vi "Sinewave_Linearity_trial_F027.vi"(0 "Array":u32[](array[numeric]), 1 "Histogram Capture Method":bool, 2 "L code":u32, 3 "UCode":dbl, 4 "Resolution":i64, 5 "Histogram: h(x)":i32[](array[numeric])) -> (6 "Average Hits \nper Code":dbl format="%.2f", 7 "Max\nDNL":dbl format="%.2f", 8 "Min\nDNL":dbl format="%.2f", 9 "Max\nINL":dbl format="%.2f", 10 "Min\nINL":dbl format="%.2f", 11 "Missing Codes":i32[](array[numeric]), 12 "Max  DNL Loc.":i32[](array[numeric]), 13 "Min DNL Loc.":i32[](array[numeric]), 14 "Max  INL Loc":i32[](array[numeric]), 15 "Min INL Loc":i32[](array[numeric]), 16 "Histogram Plot":dbl[][](graph), 17 "DNL Plot":dbl[](graph), 18 "INL Plot":dbl[](graph))   [LabVIEW 2021]
uses:
  <vilib>/Analysis/baseanly.llb/Mean (DBL).vi
  <vilib>/Analysis/NI_AALBase.lvlib
panel:
  out "range":dbl
  out "Histogram 2":dbl[](graph)
  out "2^x":dbl
  out "UCode 2":dbl
  out "L code 2":u32
  out "PI/Total no of sample":dbl
  in  "Ramp/Sine":bool
  out "Histogram raw data":i32[](graph)
  in  "Tab Control":enum32{"Histogram", "INL and DNL"}(tab)
  out "Histogram":i32[](graph)
  in  "?":bool=TRUE
  in  "?":bool
  in  "Help":bool
  in  "?":bool
  in  "file path":path
  in  "error in (not an error)":errorcluster
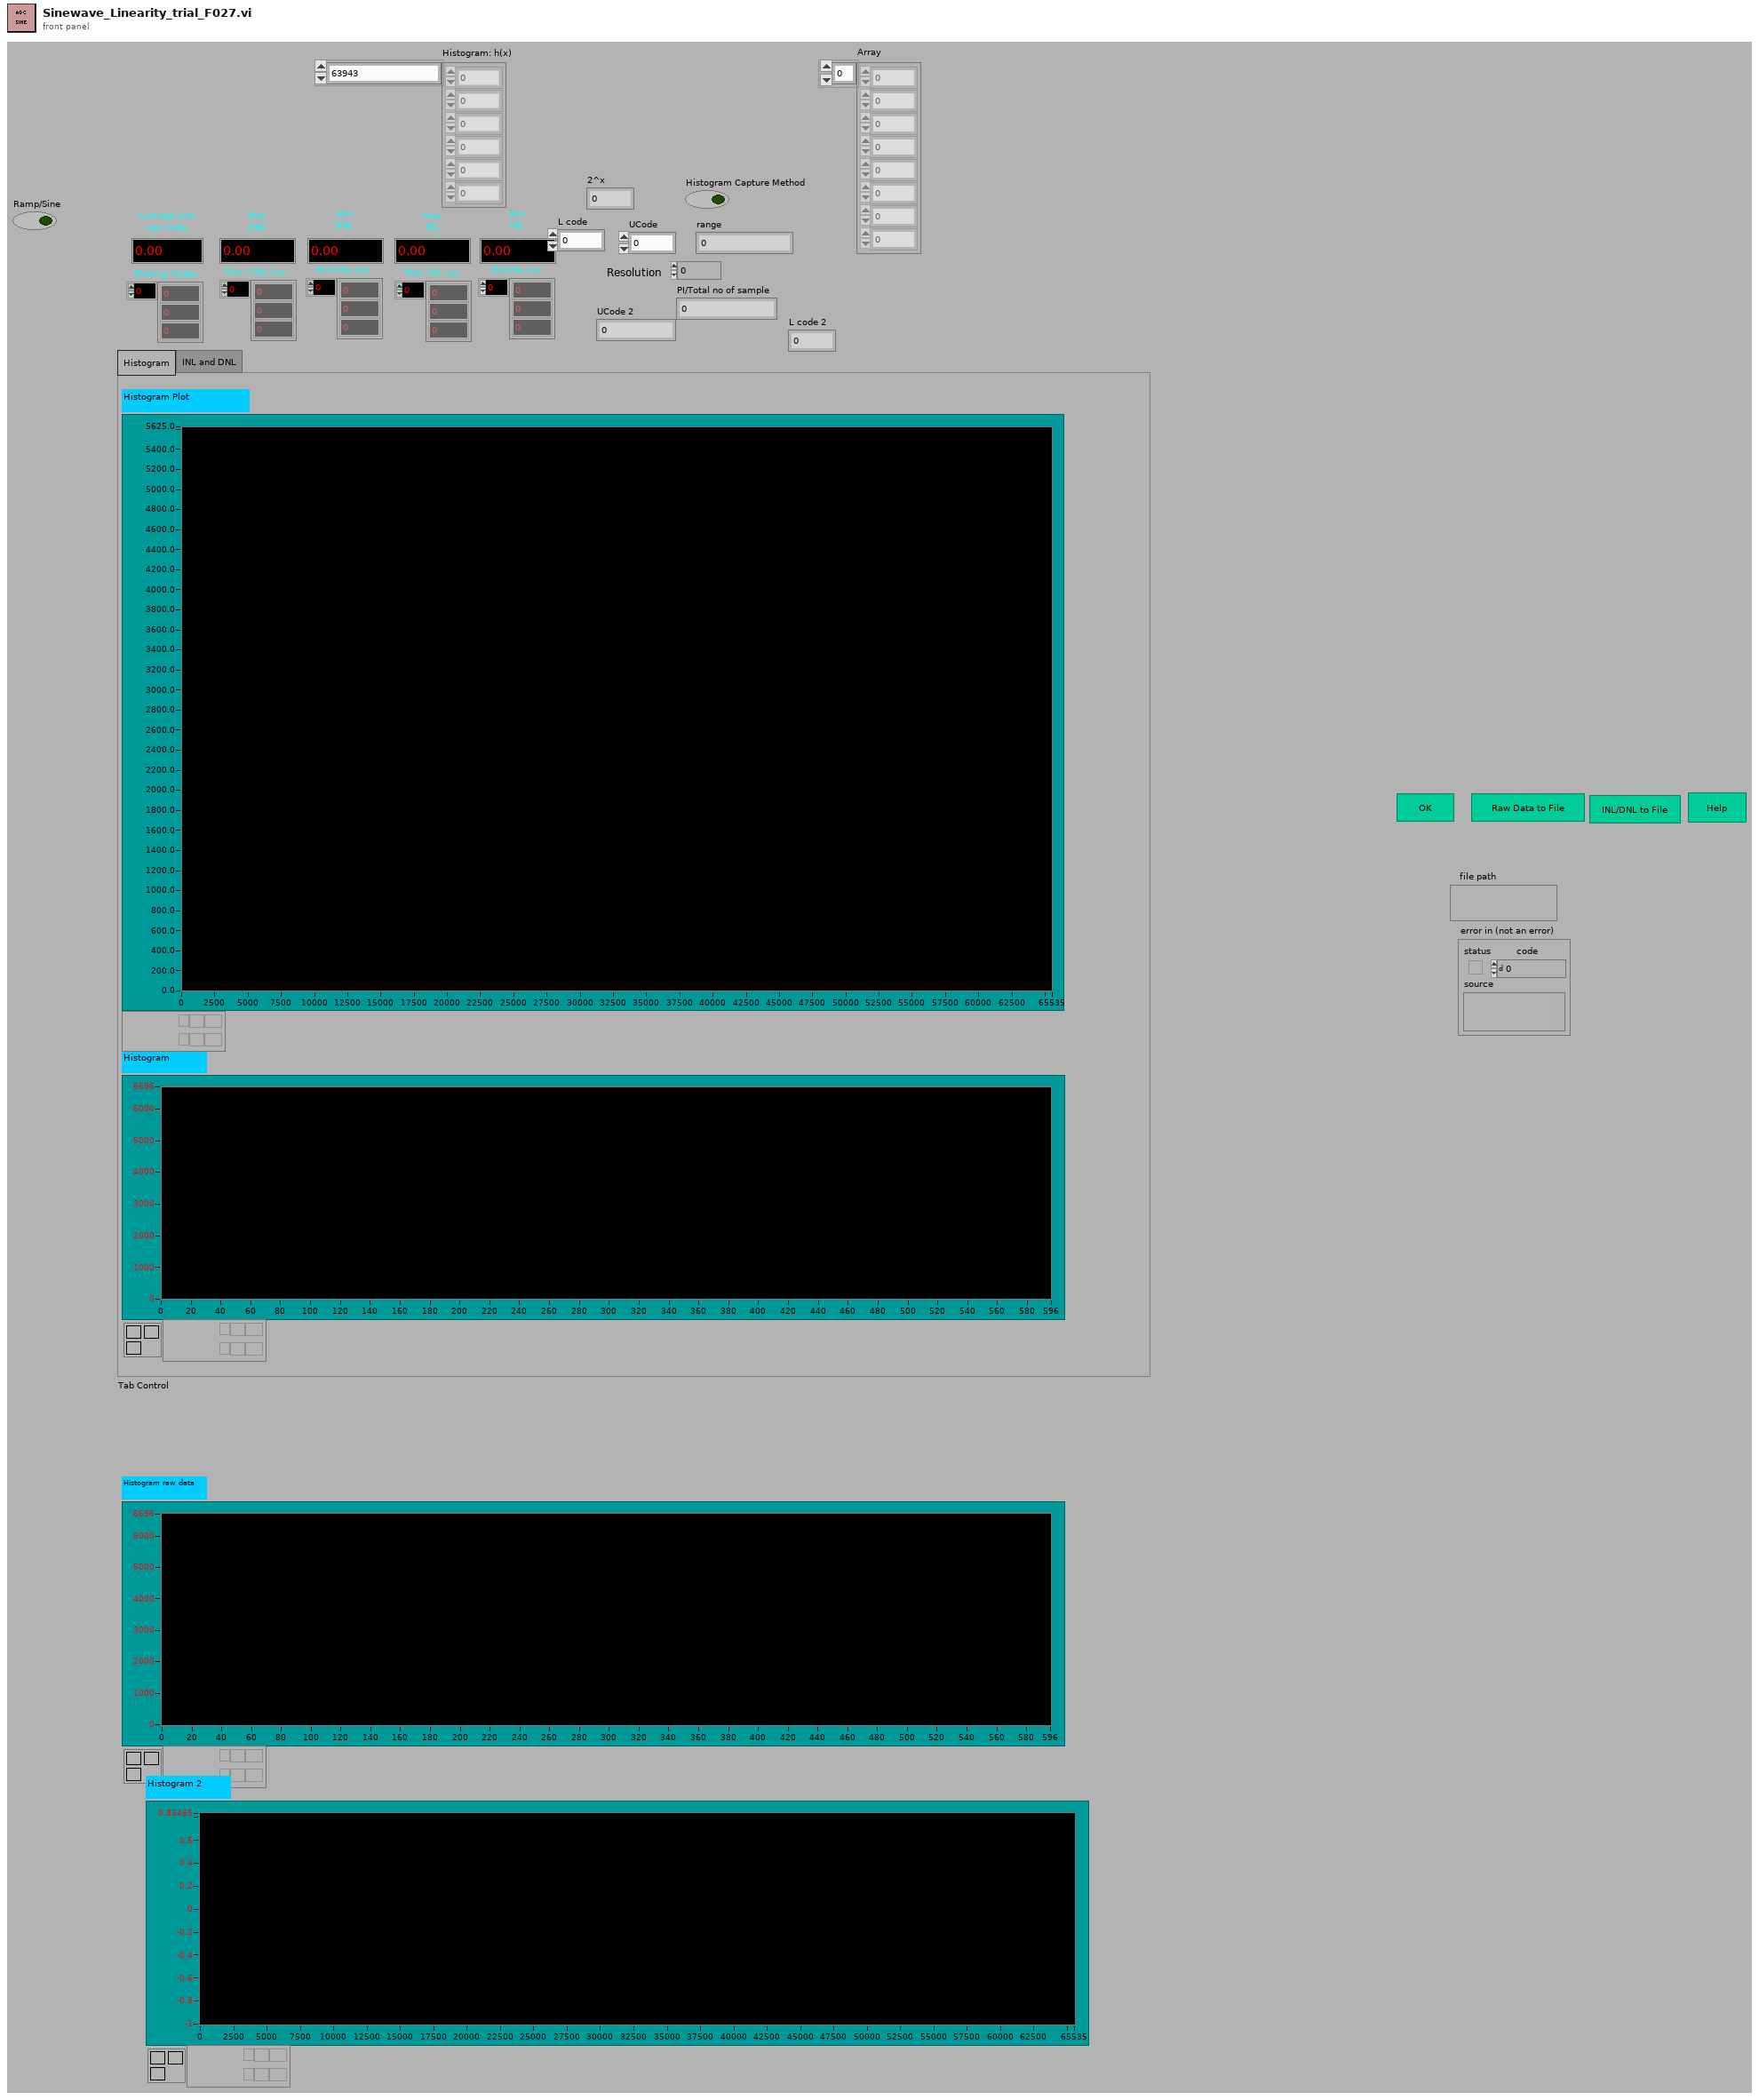
[diagram p1: front panel]
types:
  T1 = enum16{"open", "open or create", "create or replace", "create"}
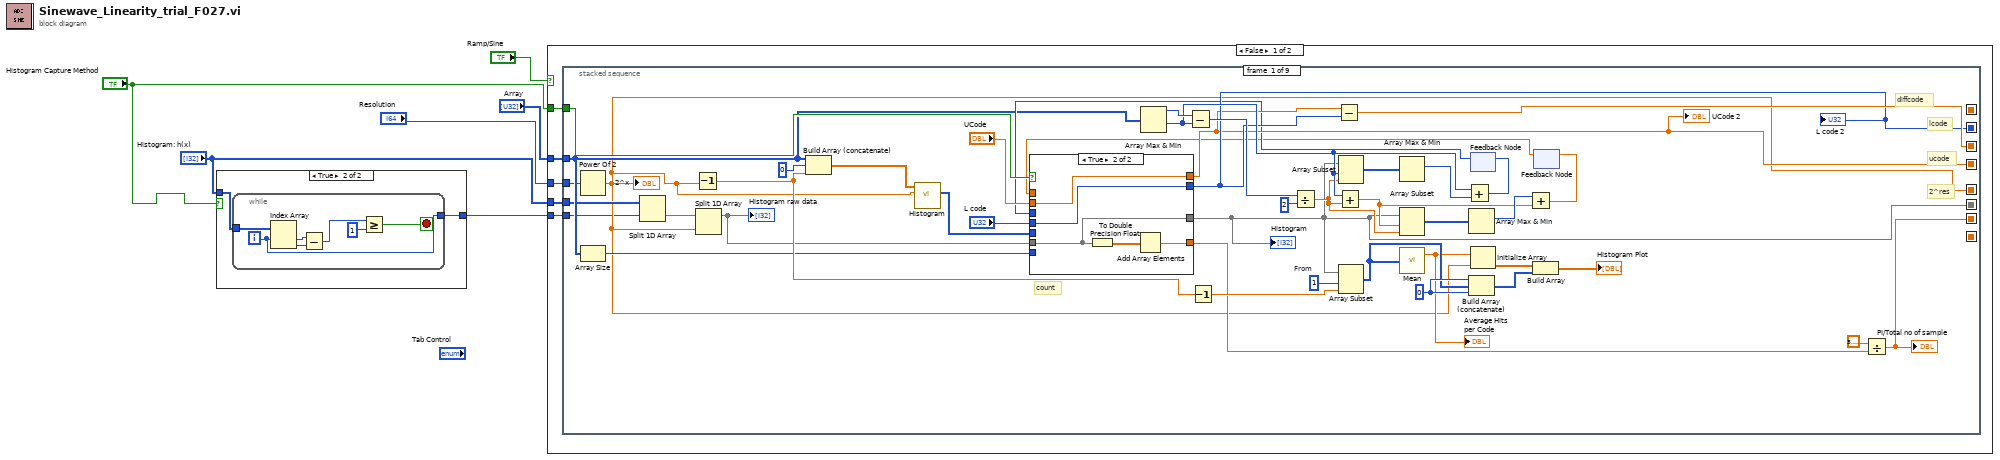
[diagram p0: block diagram]
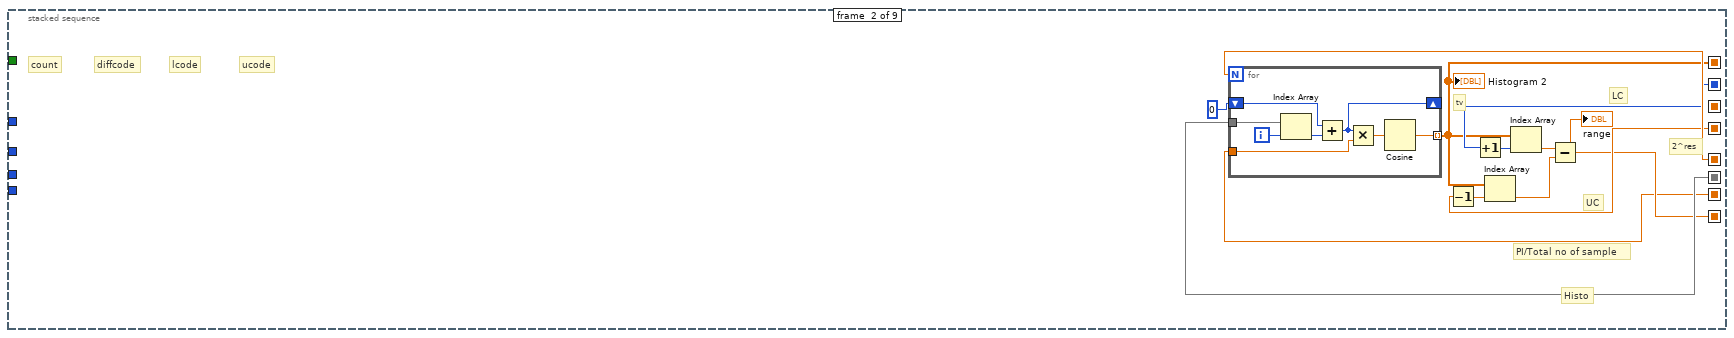
[diagram p4: hidden frame]
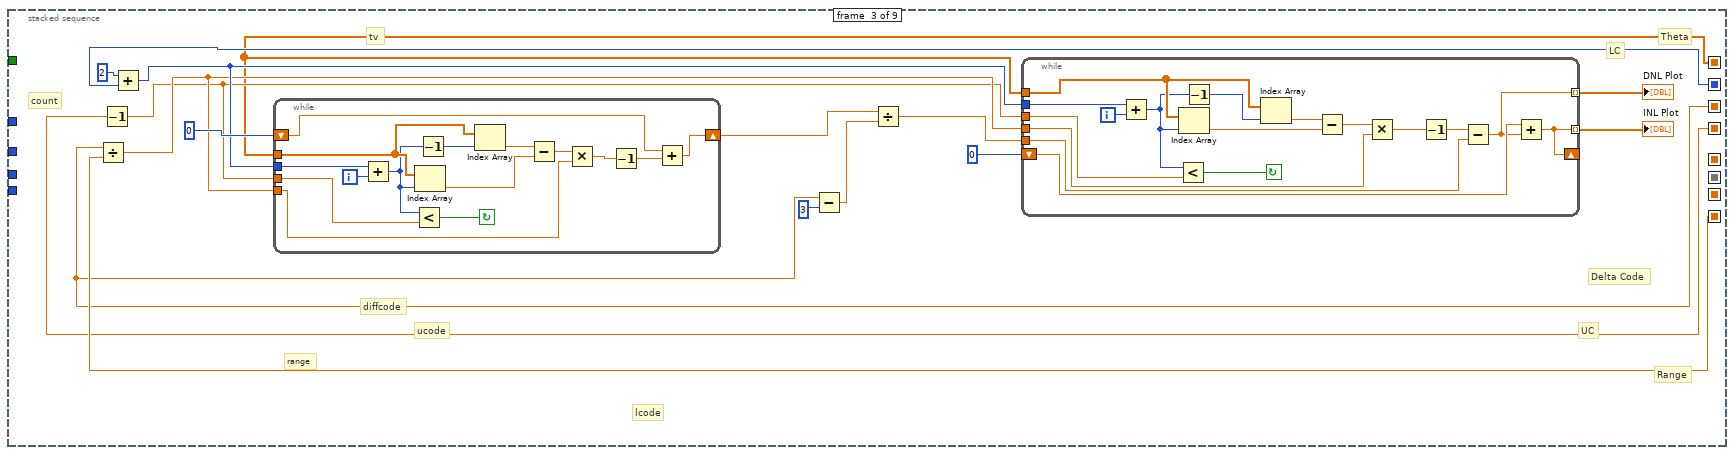
[diagram p5: hidden frame]
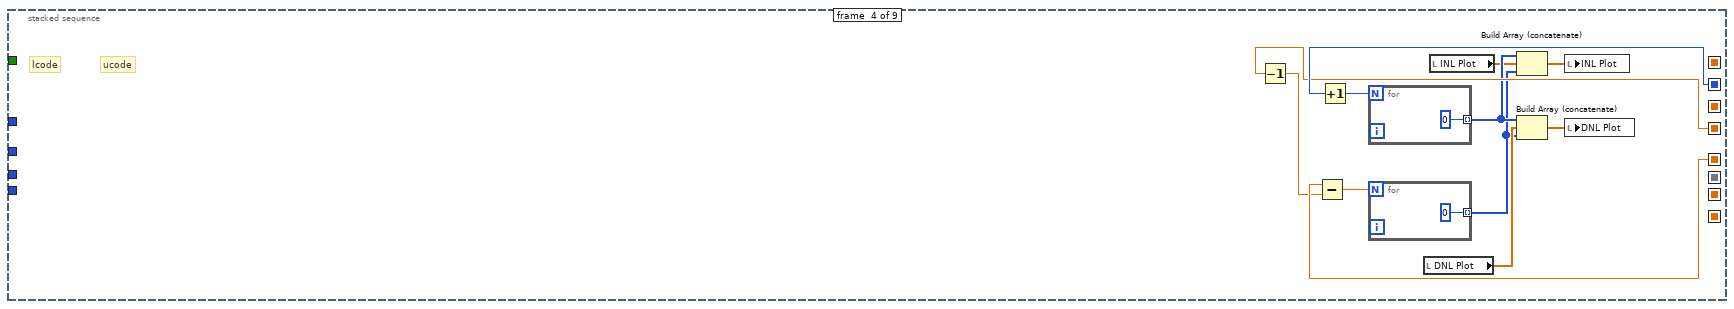
[diagram p6: hidden frame]
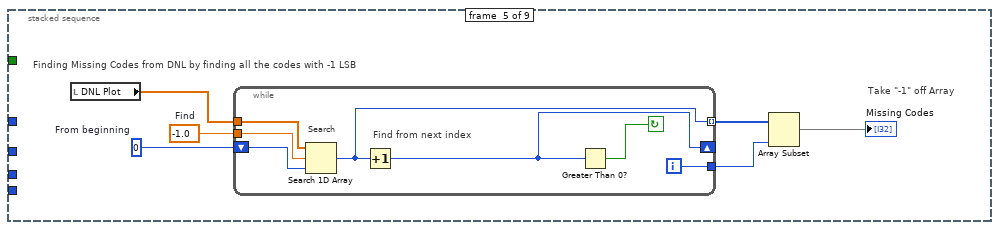
[diagram p7: hidden frame]
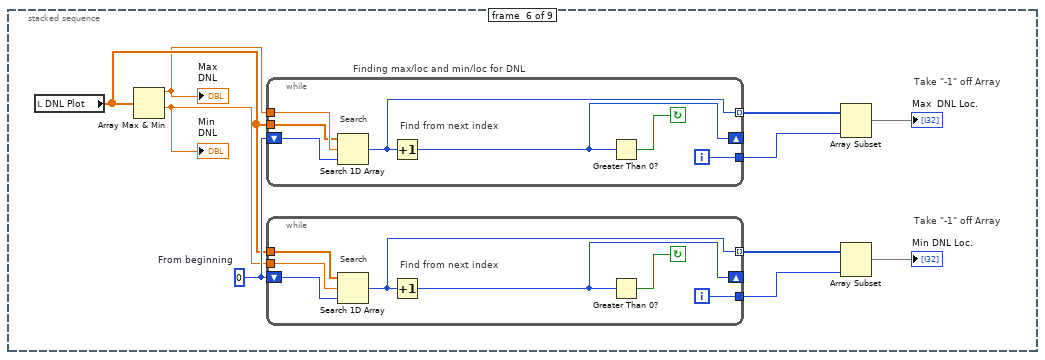
[diagram p8: hidden frame]
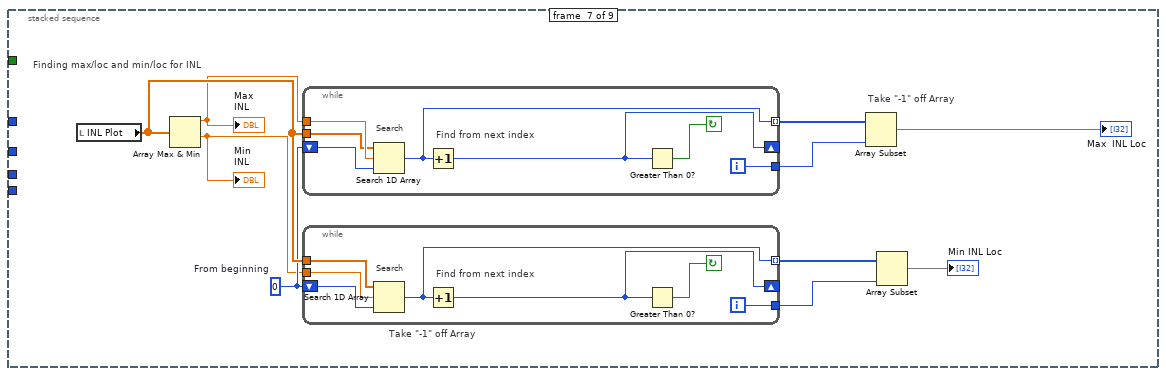
[diagram p9: hidden frame]
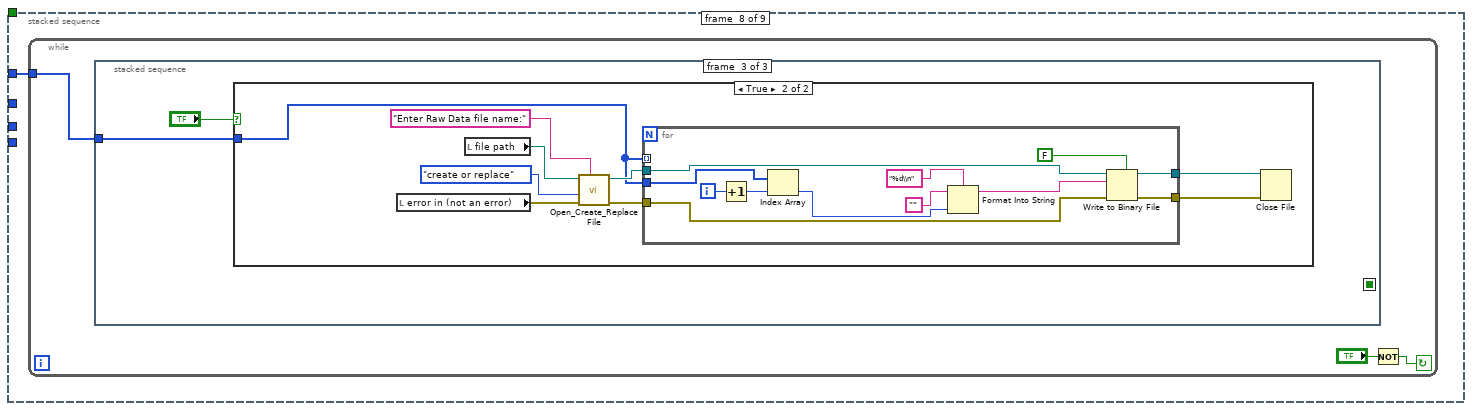
[diagram p10: hidden frame]
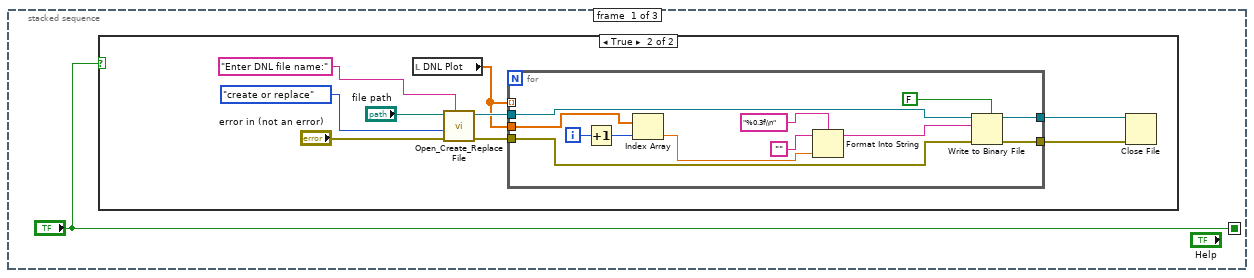
[diagram p11: hidden frame]
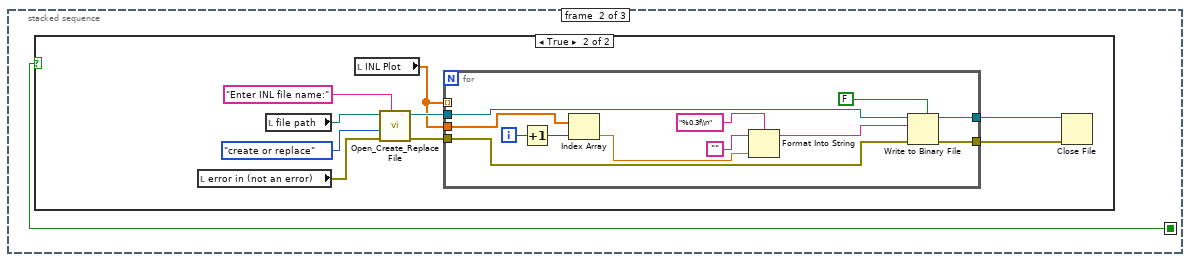
[diagram p13: hidden frame]
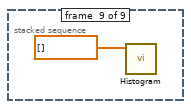
[diagram p16: hidden frame]
diagram:
  n1 = case shown="True" "Histogram Capture Method" {
    tunnel: "Histogram: h(x)" -> [_ w8]
    tunnel: [_ w7] -> w4
    frame False {
    }
    frame True {
      n2 = while {
        tunnel: w8 -> [w11]
        tunnel: [w12] -> w7
        i -> [w12]
        stop <- w14 stop-if-true
        n3 = Index Array(array=w11, index #1=w12) -> (element #1=w9:i32, element #2=w10:i32)  [unwired: 1 in]
        n4 = Subtract(x=w9, y=w10) -> (x-y=w13:i32)
        n5 = Greater Or Equal?(x=w13, y=1) -> (x >= y?=w14:bool)
      }
    }
  }
  n6 = case shown="False" "Ramp/Sine" {
    tunnel: "Resolution" -> [w20 _]
    tunnel: "Array" -> [w19 _]
    tunnel: "Histogram Capture Method" -> [w18 _]
    tunnel: "Histogram: h(x)" -> [w17 _]
    tunnel: w4 -> [w16 _]
    frame False {
      n7 = stacked-sequence {
        seq-local: [w25 _ _ _ _ _ _ _ _] -> [_ w85 _ w152 _ _ _ _ _]
        seq-local: [w21 _ _ _ _ _ _ _ _] -> [_ w83 _ _ _ _ _ _ _]
        seq-local: [w38 _ _ _ _ _ _ _ _] -> [_ w80 w103 w153 _ _ _ _ _]
        seq-local: [w37 _ _ _ _ _ _ _ _] -> [_ w79 w97 w151 _ _ _ _ _]
        seq-local: [_ w74 _ _ _ _ _ _ _] -> [_ _ w94 _ _ _ _ _ _]
        seq-local: [w51 _ _ _ _ _ _ _ _] -> [_ _ w107 _ _ _ _ _ _]
        seq-local: [_ w76 _ _ _ _ _ _ _] -> [_ _ w108 _ _ _ _ _ _]
        seq-local: [w30 _ _ _ _ _ _ _ _] -> [_ w75 _ _ _ _ _ _ _]
        tunnel: w20 -> [w26 _ _ _ _ _ _ _ _]
        tunnel: w19 -> [w33 _ _ _ _ _ _ w218 _]
        tunnel: w18 -> [w42 _ _ _ _ _ _ _ _]
        tunnel: w17 -> [w29 _ _ _ _ _ _ _ _]
        tunnel: w16 -> [w24 _ _ _ _ _ _ _ _]
        frame #0 {
          w62 = 0
          w64 = 1  # From
          # "2^res"
          # "diffcode"
          # "ucode"
          # "count"
          # "lcode"
          n8 = Power Of 2(x=w26) -> (2^x=w25:dbl)
          "2^x" <- w25
          n9 = Array Size(array=w33) -> (size(s)=w32:i32)
          n10 = Split 1D Array(array=w29, index=w24) -> (second subarray=w28:i32[])  [unwired: 1 out]
          n11 = Decrement(x=w25) -> (x-1=w55:dbl)
          n12 = Split 1D Array(array=w28, index=w25) -> (first subarray=w27:i32[])  [unwired: 1 out]
          "Histogram raw data" <- w27
          n13 = Build Array (concatenate) "Build Array"(w33, 0, w55) -> (w43:dbl[])
          n14 = call <vilib>:"Histogram.vi"("intervals"=w25, "X"=w43) -> ("Histogram: h(x)"=w41:i32[])  [unwired: 6 in, 3 out]
          n15 = Array Max & Min(array=w33) -> (max value=w49:u32, min value=w46:u32)  [unwired: 2 out]
          n16 = Subtract(x=w49, y=w46) -> (x-y=w48:u32)
          n17 = Decrement(x=w55) -> (x-1=w61:dbl)
          n18 = Divide(x=w48, y=2) -> (x/y=w45:dbl)
          n19 = Add(x=w46, y=w45) -> (x+y=w44:dbl)
          n20 = feedback #1() -> (w35:u32)  [unwired: 1 in]
          n21 = feedback #2() -> (w22:dbl)  [unwired: 1 in]
          n22 = case shown="True" w42 {
            tunnel: w41 -> [w68 _]
            tunnel: [w68 w70] -> w21
            tunnel: w27 -> [_ w70]
            tunnel: "L code" -> [_ w73]
            tunnel: "UCode" -> [_ w72]
            tunnel: [w67 w73] -> w38
            tunnel: [w66 w72] -> w37
            tunnel: w35 -> [w67 _]
            tunnel: w22 -> [w66 _]
            tunnel: w32 -> [w65 _]
            tunnel: [w65 w71] -> w31
            frame False {
            }
            frame True {
              n23 = To Double Precision Float(number=w70) -> (double precision float=w69:dbl[])
              n24 = Add Array Elements(numeric array=w69) -> (sum=w71:dbl)
            }
          }
          "Histogram" <- w21
          "L code 2" <- w38
          "UCode 2" <- w37
          n25 = Subtract(x=w37, y=w38) -> (x-y=w51:dbl)
          n26 = Array Subset(array=w21, index=w46, length=w45) -> (w53:i32[])
          n27 = Array Subset ("[1:4094]")(array=w21, index=w64, length=w61) -> (w60:i32[])
          n28 = Array Max & Min(array=w53) -> (max index (indices)=w47:i32)  [unwired: 3 out]
          n29 = Array Subset(array=w21, index=w44, length=w45) -> (w52:i32[])
          n30 = call-poly <vilib>:"Mean.vi"("X"=w60) -> ("mean"=w56:dbl)  [unwired: 1 out]
          "Average Hits \nper Code" <- w56
          n31 = Add(x=w46, y=w47) -> (x+y=w36:u32)
          n32 = Array Max & Min(array=w52) -> (max index (indices)=w50:i32)  [unwired: 3 out]
          n33 = Build Array (concatenate)(w62, w60, w62) -> (w59:i32[])
          n34 = feedback-in #1(w36) -> ()
          n35 = Initialize Array(w56, w25) -> (w58:dbl[])
          n36 = Add(x=w50, y=w44) -> (x+y=w23:dbl)
          n37 = Build Array(w58, w59) -> (→"Histogram Plot":dbl[][])
          n38 = feedback-in #2(w23) -> ()
          n39 = Divide(x=3.141592653589793, y=w31) -> (x/y=w30:dbl)
          "PI/Total no of sample" <- w30
        }
        frame #1 {
          # "LC"
          # "UC"
          # "2^res"
          # "PI/Total no of sample"
          # "Histo"
          # "diffcode"
          # "tv"
          # "ucode"
          # "count"
          # "lcode"
          n40 = for {
            N: w85 -> [_]
            shift-right: [w89] -> _
            shift-left: 0 -> [w90]
            tunnel: w83 -> [w92]
            tunnel: w75 -> [w88]
            tunnel: [w86] -> w74 mode=indexing
            i -> [w93]
            n41 = Index Array(array=w92, index=w93) -> (element=w91:i32)
            n42 = Add(x=w90, y=w91) -> (x+y=w89:i32)
            n43 = Multiply(x=w89, y=w88) -> (x*y=w87:dbl)
            n44 = Cosine(x=w87) -> (cos(x)=w86:dbl)
          }
          "Histogram 2" <- w74
          n45 = Decrement(x=w79) -> (x-1=w81:dbl)
          n46 = Increment(x=w80) -> (x+1=w82:u32)
          n47 = Index Array(array=w74, index=w81) -> (element=w77:dbl)
          n48 = Index Array(array=w74, index=w82) -> (element=w78:dbl)
          n49 = Subtract(x=w78, y=w77) -> (x-y=w76:dbl)
          "range" <- w76
        }
        frame #2 {
          # "UC"
          # "Delta Code"
          # "LC"
          # "Theta"
          # "Range"
          # "range"
          # "diffcode"
          # "tv"
          # "ucode"
          # "count"
          # "lcode"
          n50 = Divide(x=w107, y=w108) -> (x/y=w100:dbl)
          n51 = Decrement(x=w97) -> (x-1=w98:dbl)
          n52 = Add(x=2, y=w103) -> (x+y=w102:u32)
          n53 = while {
            tunnel: w100 -> [w115]
            tunnel: w94 -> [w121]
            shift-left: 0 -> [w112]
            shift-right: [w111] -> w104
            tunnel: w98 -> [w122]
            tunnel: w102 -> [w124]
            i -> [w125]
            stop <- w123 continue-if-true
            n54 = Add(x=w124, y=w125) -> (x+y=w119:u32)
            n55 = Less?(x=w119, y=w122) -> (x < y?=w123:bool)
            n56 = Index Array(array=w121, index=w119) -> (element=w117:dbl)
            n57 = Decrement(x=w119) -> (x-1=w120:u32)
            n58 = Index Array(array=w121, index=w120) -> (element=w118:dbl)
            n59 = Subtract(x=w118, y=w117) -> (x-y=w116:dbl)
            n60 = Multiply(x=w116, y=w115) -> (x*y=w114:dbl)
            n61 = Decrement(x=w114) -> (x-1=w113:dbl)
            n62 = Add(x=w112, y=w113) -> (x+y=w111:dbl)
          }
          n63 = Subtract(x=w107, y=3) -> (x-y=w105:dbl)
          n64 = Divide(x=w104, y=w105) -> (x/y=w99:dbl)
          n65 = while {
            tunnel: [w126] -> w95 mode=indexing
            tunnel: [w127] -> w96 mode=indexing
            tunnel: w99 -> [w128]
            tunnel: w100 -> [w132]
            tunnel: w94 -> [w138]
            shift-left: 0 -> [w130]
            shift-right: [w126] -> _
            tunnel: w98 -> [w139]
            tunnel: w102 -> [w141]
            i -> [w142]
            stop <- w140 continue-if-true
            n66 = Add(x=w141, y=w142) -> (x+y=w136:u32)
            n67 = Less?(x=w136, y=w139) -> (x < y?=w140:bool)
            n68 = Index Array(array=w138, index=w136) -> (element=w134:dbl)
            n69 = Decrement(x=w136) -> (x-1=w137:u32)
            n70 = Index Array(array=w138, index=w137) -> (element=w135:dbl)
            n71 = Subtract(x=w135, y=w134) -> (x-y=w133:dbl)
            n72 = Multiply(x=w133, y=w132) -> (x*y=w131:dbl)
            n73 = Decrement(x=w131) -> (x-1=w129:dbl)
            n74 = Subtract(x=w129, y=w128) -> (x-y=w127:dbl)
            n75 = Add(x=w130, y=w127) -> (x+y=w126:dbl)
          }
          "DNL Plot" <- w96
          "INL Plot" <- w95
        }
        frame #3 {
          # "ucode"
          # "lcode"
          n76 = Decrement(x=w151) -> (x-1=w145:dbl)
          n77 = Subtract(x=w152, y=w145) -> (x-y=w150:dbl)
          n78 = Increment(x=w153) -> (x+1=w154:u32)
          n79 = for {
            N: w154 -> [_]
            tunnel: [0] -> w148 mode=indexing
          }
          n80 = for {
            N: w150 -> [_]
            tunnel: [0] -> w147 mode=indexing
          }
          n81 = local read "DNL Plot"() -> (w149:dbl[])
          n82 = local read "INL Plot"() -> (w146:dbl[])
          n83 = Build Array (concatenate)(w148, w146, w147) -> (w143:dbl[])
          n84 = Build Array (concatenate)(w148, w149, w147) -> (w144:dbl[])
          n85 = local write "INL Plot"(w143) -> ()
          n86 = local write "DNL Plot"(w144) -> ()
        }
        frame #4 {
          w161 = 0  # From beginning
          w162 = -1.0  # Find
          # "Take \"-1\" off Array"
          # "Finding Missing Codes from DNL by finding all the codes with -1 LSB"
          n87 = local read "DNL Plot"() -> (w158:dbl[])
          n88 = while {
            tunnel: [w163] -> w159
            tunnel: [w164] -> w160 mode=indexing
            tunnel: w158 -> [w167]
            tunnel: w162 -> [w168]
            shift-left: w161 -> [w169]
            shift-right: [w166] -> _
            i -> [w163]
            stop <- w165 continue-if-true
            # "Search"
            # "Find from next index"
            n89 = Search 1D Array(1D array=w167, element=w168, start index (0)=w169) -> (index of element=w164:i32)
            n90 = Increment(x=w164) -> (x+1=w166:i32)
            n91 = Greater Than 0?(x=w166) -> (x > 0?=w165:bool)
          }
          n92 = Array Subset(array=w160, length=w159) -> (→"Missing Codes":i32[])  [unwired: 1 in]
        }
        frame #5 {
          w179 = 0  # From beginning
          # "Finding max/loc and min/loc for DNL"
          # "Take \"-1\" off Array"
          # "Take \"-1\" off Array"
          n93 = local read "DNL Plot"() -> (w178:dbl[])
          n94 = Array Max & Min(array=w178) -> (max value=w171:dbl, min value=w170:dbl)  [unwired: 2 out]
          "Min\nDNL" <- w170
          "Max\nDNL" <- w171
          n95 = while {
            tunnel: w178 -> [w187]
            tunnel: w171 -> [w188]
            tunnel: [w189] -> w175 mode=indexing
            tunnel: [w190] -> w174
            shift-left: w179 -> [w193]
            shift-right: [w192] -> _
            i -> [w190]
            stop <- w191 continue-if-true
            # "Search"
            # "Find from next index"
            n96 = Search 1D Array(1D array=w187, element=w188, start index (0)=w193) -> (index of element=w189:i32)
            n97 = Increment(x=w189) -> (x+1=w192:i32)
            n98 = Greater Than 0?(x=w192) -> (x > 0?=w191:bool)
          }
          n99 = while {
            tunnel: w178 -> [w180]
            tunnel: w170 -> [w181]
            tunnel: [w182] -> w177 mode=indexing
            tunnel: [w183] -> w176
            shift-left: w179 -> [w186]
            shift-right: [w185] -> _
            i -> [w183]
            stop <- w184 continue-if-true
            # "Search"
            # "Find from next index"
            n100 = Search 1D Array(1D array=w180, element=w181, start index (0)=w186) -> (index of element=w182:i32)
            n101 = Increment(x=w182) -> (x+1=w185:i32)
            n102 = Greater Than 0?(x=w185) -> (x > 0?=w184:bool)
          }
          n103 = Array Subset(array=w175, length=w174) -> (→"Max  DNL Loc.":i32[])  [unwired: 1 in]
          n104 = Array Subset(array=w177, length=w176) -> (→"Min DNL Loc.":i32[])  [unwired: 1 in]
        }
        frame #6 {
          w198 = 0  # From beginning
          # "Take \"-1\" off Array"
          # "Take \"-1\" off Array"
          # "Finding max/loc and min/loc for INL"
          n105 = local read "INL Plot"() -> (w199:dbl[])
          n106 = Array Max & Min(array=w199) -> (max value=w197:dbl, min value=w196:dbl)  [unwired: 2 out]
          "Max\nINL" <- w197
          "Min\nINL" <- w196
          n107 = while {
            tunnel: w199 -> [w204]
            tunnel: w197 -> [w205]
            tunnel: [w206] -> w202 mode=indexing
            tunnel: [w207] -> w203
            shift-left: w198 -> [w210]
            shift-right: [w209] -> _
            i -> [w207]
            stop <- w208 continue-if-true
            # "Search"
            # "Find from next index"
            n108 = Search 1D Array(1D array=w204, element=w205, start index (0)=w210) -> (index of element=w206:i32)
            n109 = Increment(x=w206) -> (x+1=w209:i32)
            n110 = Greater Than 0?(x=w209) -> (x > 0?=w208:bool)
          }
          n111 = while {
            tunnel: w199 -> [w211]
            tunnel: w196 -> [w212]
            tunnel: [w213] -> w200 mode=indexing
            tunnel: [w214] -> w201
            shift-left: w198 -> [w217]
            shift-right: [w216] -> _
            i -> [w214]
            stop <- w215 continue-if-true
            # "Search"
            # "Find from next index"
            n112 = Search 1D Array(1D array=w211, element=w212, start index (0)=w217) -> (index of element=w213:i32)
            n113 = Increment(x=w213) -> (x+1=w216:i32)
            n114 = Greater Than 0?(x=w216) -> (x > 0?=w215:bool)
          }
          n115 = Array Subset(array=w202, length=w203) -> (→"Max  INL Loc":i32[])  [unwired: 1 in]
          n116 = Array Subset(array=w200, length=w201) -> (→"Min INL Loc":i32[])  [unwired: 1 in]
        }
        frame #7 {
          n117 = while {
            tunnel: w218 -> [w219]
            stop <- w220 continue-if-true
            n118 = stacked-sequence {
              seq-local: ["?" _ _] -> [_ w244 _]
              tunnel: w219 -> [_ _ w266]
              frame #0 {
                n119 = case shown="True" "?" {
                  frame False {
                  }
                  frame True {
                    n120 = local read "DNL Plot"() -> (w228:dbl[])
                    n121 = call <vilib>:"Open_Create_Replace File.vi"("prompt"="Enter DNL file name:", "error in (no error)"="error in (not an error)", "function (open:0)"=T1."create or replace", "file path"="file path") -> ("error out"=w229:errorcluster, "refnum"=w230:refnum<file>)  [unwired: 4 in, 2 out]
                    n122 = for {
                      tunnel: w228 -> [w240]
                      tunnel: w230 -> [w238]
                      tunnel: w229 -> [w237]
                      tunnel: [w236] -> w227
                      tunnel: [w235] -> w226
                      tunnel: w228 -> [_] mode=indexing
                      i -> [w234]
                      n123 = Increment(x=w234) -> (x+1=w233:i32)
                      n124 = Index Array(array=w240, index=w233) -> (element=w241:dbl)
                      n125 = Format Into String(format string="%0.3f\\n", initial string="", w241) -> (resulting string=w239:string)  [unwired: 1 in, 1 out]
                      n126 = Write to Binary File(file (use dialog)=w238, data=w239, error in=w237, 5:FALSE ("prepend array or string size? (T)")) -> (refnum out=w236:refnum<file>, error out=w235:errorcluster)  [unwired: 2 in, 1 out]
                    }
                    n127 = Close File(refnum=w227, error in=w226) -> ()  [unwired: 2 out]
                  }
                }
              }
              frame #1 {
                n128 = case shown="True" w244 {
                  frame False {
                  }
                  frame True {
                    n129 = local read "error in (not an error)"() -> (w245:errorcluster)
                    n130 = local read "file path"() -> (w246:path)
                    n131 = local read "INL Plot"() -> (w250:dbl[])
                    n132 = call <vilib>:"Open_Create_Replace File.vi"("prompt"="Enter INL file name:", "error in (no error)"=w245, "function (open:0)"=T1."create or replace", "file path"=w246) -> ("error out"=w251:errorcluster, "refnum"=w252:refnum<file>)  [unwired: 4 in, 2 out]
                    n133 = for {
                      tunnel: w250 -> [w262]
                      tunnel: w252 -> [w260]
                      tunnel: w251 -> [w259]
                      tunnel: [w258] -> w249
                      tunnel: [w257] -> w248
                      tunnel: w250 -> [_] mode=indexing
                      i -> [w256]
                      n134 = Increment(x=w256) -> (x+1=w255:i32)
                      n135 = Index Array(array=w262, index=w255) -> (element=w263:dbl)
                      n136 = Format Into String(format string="%0.3f\\n", initial string="", w263) -> (resulting string=w261:string)  [unwired: 1 in, 1 out]
                      n137 = Write to Binary File(file (use dialog)=w260, data=w261, error in=w259, 5:FALSE ("prepend array or string size? (T)")) -> (refnum out=w258:refnum<file>, error out=w257:errorcluster)  [unwired: 2 in, 1 out]
                    }
                    n138 = Close File(refnum=w249, error in=w248) -> ()  [unwired: 2 out]
                  }
                }
              }
              frame #2 {
                n139 = case shown="True" "?" {
                  tunnel: w266 -> [_ w268]
                  frame False {
                  }
                  frame True {
                    n140 = local read "error in (not an error)"() -> (w269:errorcluster)
                    n141 = local read "file path"() -> (w270:path)
                    n142 = call <vilib>:"Open_Create_Replace File.vi"("prompt"="Enter Raw Data file name:", "error in (no error)"=w269, "function (open:0)"=T1."create or replace", "file path"=w270) -> ("error out"=w274:errorcluster, "refnum"=w275:refnum<file>)  [unwired: 4 in, 2 out]
                    n143 = for {
                      tunnel: w275 -> [w284]
                      tunnel: w274 -> [w283]
                      tunnel: [w282] -> w273
                      tunnel: [w281] -> w272
                      tunnel: w268 -> [w277]
                      tunnel: w268 -> [_] mode=indexing
                      i -> [w280]
                      n144 = Increment(x=w280) -> (x+1=w279:i32)
                      n145 = Index Array(array=w277, index=w279) -> (element=w286:u32)
                      n146 = Format Into String(format string="%d\\n", initial string="", w286) -> (resulting string=w285:string)  [unwired: 1 in, 1 out]
                      n147 = Write to Binary File(file (use dialog)=w284, data=w285, error in=w283, 5:FALSE ("prepend array or string size? (T)")) -> (refnum out=w282:refnum<file>, error out=w281:errorcluster)  [unwired: 2 in, 1 out]
                    }
                    n148 = Close File(refnum=w273, error in=w272) -> ()  [unwired: 2 out]
                  }
                }
              }
            }
            n149 = Not(x="?") -> (.not. x?=w220:bool)
          }
        }
        frame #8 {
          n150 = call <vilib>:"Histogram.vi"("X"=dbl[] []) -> ()  [unwired: 7 in, 4 out]
        }
      }
    }
    frame True {
    }
  }
